vi "Get Notification Handle.vi"(7 "Alias":string, 8 "error in (no error)":errorcluster, 10 "Symbol Name":string, 11 "TwinCAT ADS in":refnum<class "TwinCAT ADS.lvclass">) -> (0 "error out":errorcluster, 2 "Handle":i32, 3 "TwinCAT ADS out":refnum<class "TwinCAT ADS.lvclass">)   [LabVIEW 2018, in "TwinCAT ADS.lvclass"]
uses:
  TwinCAT ADS.lvclass
  TwinCAT ADS.lvclass/TwinCAT ADS.ctl
  Get Notification Map.vi
  To Notification Key.vi
  <vilib>/Utility/error.llb/Trim Whitespace.vi
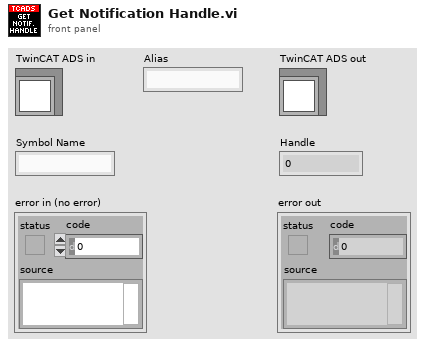
[diagram p1: front panel]
types:
  T1 = typedef "TwinCAT ADS.lvclass/Notifcation Map Value.ctl" = cluster{"Handle":i32, "Cycle Time":i32}
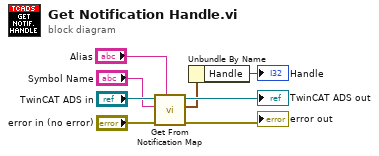
[diagram p0: block diagram]
diagram:
  n1 = call "Get From Notification Map.vi"("Alias"="Alias", "error in (no error)"="error in (no error)", "Symbol Name"="Symbol Name", "TwinCAT ADS in"="TwinCAT ADS in") -> ("error out"=→"error out":errorcluster, "Value"=w3:T1, "TwinCAT ADS out"=→"TwinCAT ADS out":refnum<class "TwinCAT ADS.lvclass">)  [unwired: 5 in]
  n2 = Unbundle By Name(w3) -> ("Handle"=→"Handle":i32)
